vi "Autonomous Independent.vi"() -> ()   [LabVIEW 2013]
doc: "This VI is called when autonomous begins, and will automatically be terminated when autonomous ends. You can carry out timed or sensor driven robot movement independently without needing to return to the caller."
uses:
  Robot Global Data.vi
  <vilib>/Rock Robotics/WPI/RobotDrive/WPI_RobotDriveMecanumDrive_Cartesian.vi
  <vilib>/Rock Robotics/WPI/RobotDrive/WPI_RobotDriveGetSetRefNum.vi
panel:
  out "Current Movement, for debugging":T1 {"Z Joystick Value" scale=-1.0..1.0; "Y Joystick Value" scale=1.0..-1.0; "X Joystick Value" scale=-1.0..1.0}
  in  "Array of robot movements":T2(array[cluster]) {"Z Joystick Value" scale=-1.0..1.0; "Y Joystick Value" scale=1.0..-1.0; "X Joystick Value" scale=-1.0..1.0}
  # "Be sure to right-click and choose Data Operations>>Make Current Value default if you want to save the array values with the VI"
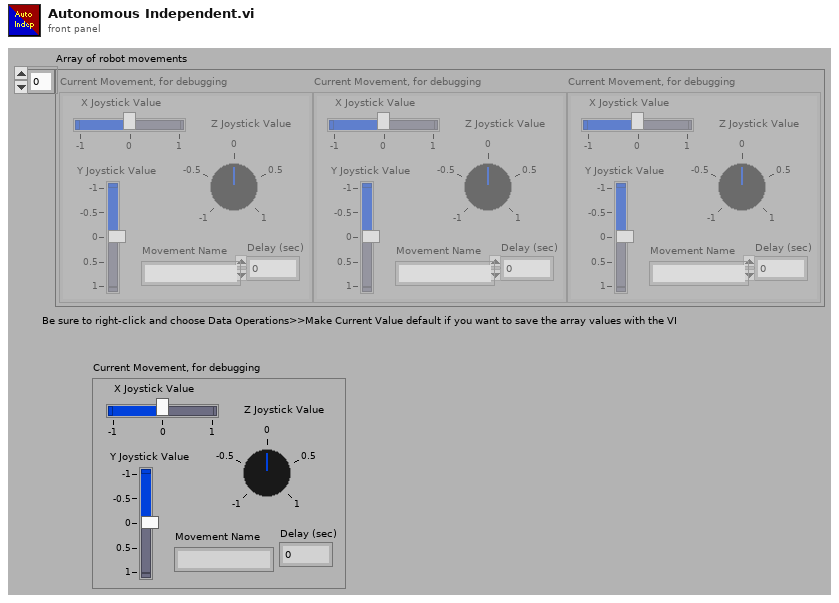
[diagram p1: front panel]
types:
  T1 = cluster{"X Joystick Value":dbl, "Y Joystick Value":dbl, "Z Joystick Value":dbl, "Delay (sec)":dbl, "Movement Name":string}
  T2 = cluster{"X Joystick Value":dbl, "Y Joystick Value":dbl, "Z Joystick Value":dbl, "Delay (sec)":dbl, "Movement Name":string}[]
  T3 = typedef "WPI_RobotDriveDevRef.ctl" = cluster{"DevStatus":errorcluster, "Motors[]":T4[], "Square Inputs":bool, "Max Output":dbl, "Isochronous":bool}
  T4 = typedef "WPI_MotorControlDeviceRef.ctl" = cluster{"DeviceStatus":errorcluster, "Type":enum16{"PWM", "CAN"}, "PWM":cluster{"Digital Module":T5, "PWM Channel":T6, "DeadBand":T7}, "CAN":cluster{"Device Number":u8, "Control Mode":T8, "Semaphore":T9, "Max Vout":dbl}, "Invert":bool, "TransformRef":T10, "InvTransformRef":T10}
  T5 = typedef "FPGA_TypedefDigitalModule.ctl" = enum16{"Digital Module 1", "Digital Module 2"}
  T6 = typedef "FPGA_DIOPWMChannel.ctl" = enum8{"PWM 1", "PWM 2", "PWM 3", "PWM 4", "PWM 5", "PWM 6", "PWM 7", "PWM 8", "PWM 9", "PWM 10", "Invalid"}
  T7 = typedef "WPI_PWMDeadband.ctl" = cluster{"Name":string, "maxPositivePwm":i32, "minPositivePwm":i32, "centerPwm":i32, "maxNegativePwm":i32, "minNegativePwm":i32, "angularRange":u16}
  T8 = typedef "WPI_CANJaguar_ControlMode.ctl" = enum8{"Percent VBus", "Current", "Speed", "Position", "Voltage"}
  T9 = typedef "Semaphore RefNum" = refnum<k1>
  T10 = typedef "WPI_PWMTransform_ConPane.ctl" = refnum<vi>
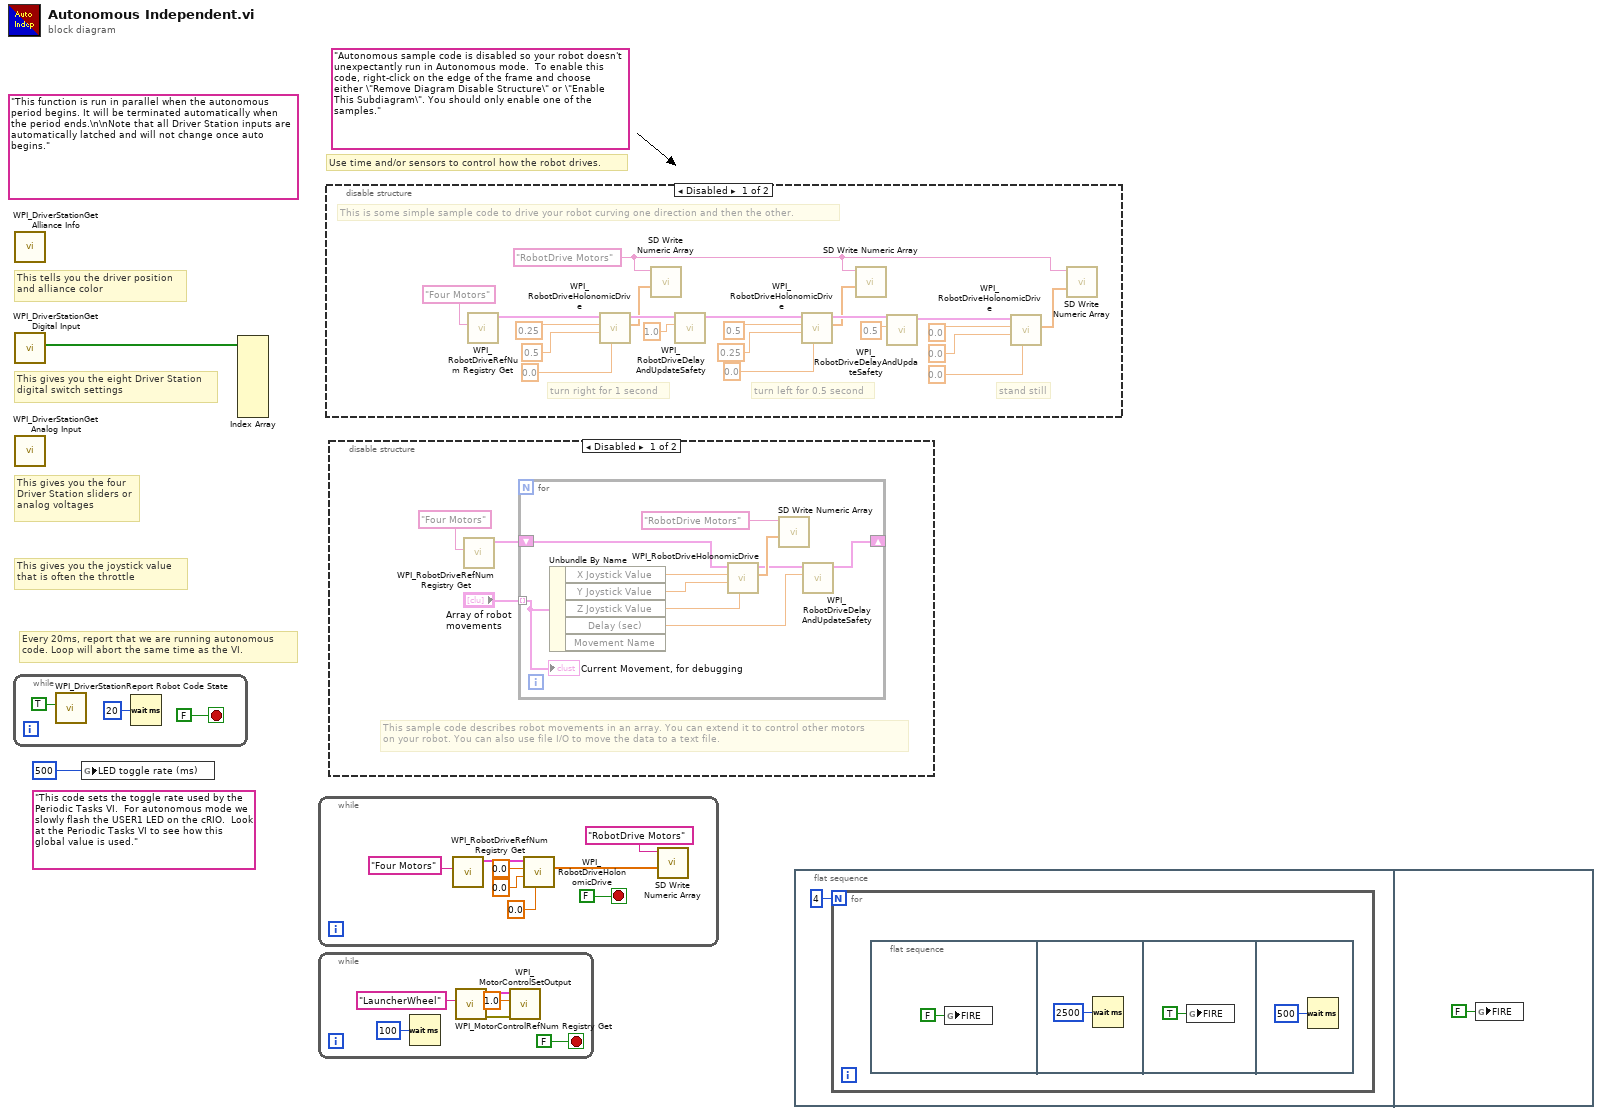
[diagram p0: block diagram]
diagram:
  (unwired) "This code sets the toggle rate used by the Periodic Tasks VI.  For autonomous mode we slowly flash the USER1 LED on the cRIO.  Look at the Periodic Tasks VI to see how this global value is used."
  (unwired) "Autonomous sample code is disabled so your robot doesn't unexpectantly run in Autonomous mode.  To enable this code, right-click on the edge of the frame and choose either \"Remove Diagram Disable Structure\" or \"Enable This Subdiagram\". You should only enable one of the samples."
  (unwired) "This function is run in parallel when the autonomous period begins. It will be terminated automatically when the period ends.\n\nNote that all Driver Station inputs are automatically latched and will not change once auto begins."
  # "Every 20ms, report that we are running autonomous\ncode. Loop will abort the same time as the VI."
  # "This gives you the joystick value\nthat is often the throttle"
  # "Use time and/or sensors to control how the robot drives."
  # "This tells you the driver position\nand alliance color"
  # "This gives you the eight Driver Station\ndigital switch settings"
  # "This gives you the four\nDriver Station sliders or\nanalog voltages"
  n1 = while {
    stop <- FALSE stop-if-true
    n2 = call <vilib>:"WPI_DriverStationReport Robot Code State.vi"("Autonomous"=TRUE) -> ()  [unwired: 10 in, 1 out]
    n3 = Wait (ms)(milliseconds to wait=u32 20) -> ()  [unwired: 1 out]
  }
  n4 = call <vilib>:"WPI_DriverStationGet Alliance Info.vi"() -> ()  [unwired: 12 out]
  n5 = call <vilib>:"WPI_DriverStationGet Digital Input.vi"() -> ("Driver Station Digital Input (1-8)"=w2:bool[])  [unwired: 11 out]
  n6 = call <vilib>:"WPI_DriverStationGet Analog Input.vi"() -> ()  [unwired: 12 out]
  n7 = global write "Robot Global Data.vi" "LED toggle rate (ms)"(u32 500 ("LED ms toggle rate")) -> ()
  n8 = Index Array(array=w2) -> ()  [unwired: 8 in, 8 out]
  n9 = while {
    stop <- FALSE stop-if-true
    n10 = call <vilib>:"WPI_RobotDriveRefNum Registry Get.vi"("refnum name"="Four Motors") -> ("RobotDriveDevRef"=w11:T3)  [unwired: 1 in, 9 out]
    n11 = call-poly <vilib>:"WPI_RobotDriveHolonomicDrive.vi"("Rotation"=0.0, "Y"=0.0, "X"=0.0, "RobotDriveDevRef"=w11) -> ("Motor Values"=w9:dbl[])  [unwired: 5 in, 2 out]
    n12 = call <vilib>:"SD Write Numeric Array.vi"("Numeric Array"=w9, "Name"="RobotDrive Motors") -> ()  [unwired: 8 in, 2 out]
  }
  n13 = while {
    stop <- FALSE stop-if-true
    n14 = Wait (ms)(milliseconds to wait=u32 100) -> ()  [unwired: 1 out]
    n15 = call <vilib>:"WPI_MotorControlRefNum Registry Get.vi"("refnum name"="LauncherWheel") -> ("error out"=w18:errorcluster, "MotorControlDevRef"=w19:T4)  [unwired: 9 in]
    n16 = call <vilib>:"WPI_MotorControlSetOutput.vi"("error in (no error)"=w18, "Output"=1.0, "MotorControlDevRef"=w19) -> ()  [unwired: 6 in, 3 out]
  }
  n17 = disable-structure shown="Disabled" {
    frame Disabled {
      w23 = "RobotDrive Motors" ("Name")
      # "This is some simple sample code to drive your robot curving one direction and then the other."
      # "stand still"
      # "turn left for 0.5 second"
      # "turn right for 1 second"
      n18 = call <vilib>:"WPI_RobotDriveRefNum Registry Get.vi"("refnum name"="Four Motors") -> ("RobotDriveDevRef"=w27:T3)  [unwired: 1 in, 9 out]
      n19 = call-poly <vilib>:"WPI_RobotDriveHolonomicDrive.vi"("Rotation"=0.0, "Y"=0.5 ("X axis value"), "X"=0.25 ("X axis value"), "RobotDriveDevRef"=w27) -> ("Motor Values"=w26:dbl[], "RobotDriveDevRef"=w34:T3)  [unwired: 5 in, 1 out]
      n20 = call <vilib>:"SD Write Numeric Array.vi"("Numeric Array"=w26, "Name"=w23) -> ()  [unwired: 8 in, 2 out]
      n21 = call <vilib>:"WPI_RobotDriveDelayAndUpdateSafety.vi"("Delay (s)"=1.0, "RobotDriveDevRef"=w34) -> ("RobotDriveDevRef 2"=w33:T3)  [unwired: 8 in, 1 out]
      n22 = call-poly <vilib>:"WPI_RobotDriveHolonomicDrive.vi"("Rotation"=0.0, "Y"=0.25 ("X axis value"), "X"=0.5 ("X axis value"), "RobotDriveDevRef"=w33) -> ("Motor Values"=w25:dbl[], "RobotDriveDevRef"=w32:T3)  [unwired: 5 in, 1 out]
      n23 = call <vilib>:"SD Write Numeric Array.vi"("Numeric Array"=w25, "Name"=w23) -> ()  [unwired: 8 in, 2 out]
      n24 = call <vilib>:"WPI_RobotDriveDelayAndUpdateSafety.vi"("Delay (s)"=0.5, "RobotDriveDevRef"=w32) -> ("RobotDriveDevRef 2"=w31:T3)  [unwired: 8 in, 1 out]
      n25 = call-poly <vilib>:"WPI_RobotDriveHolonomicDrive.vi"("Rotation"=0.0 ("X axis value"), "Y"=0.0 ("X axis value"), "X"=0.0 ("X axis value"), "RobotDriveDevRef"=w31) -> ("Motor Values"=w24:dbl[])  [unwired: 5 in, 2 out]
      n26 = call <vilib>:"SD Write Numeric Array.vi"("Numeric Array"=w24, "Name"=w23) -> ()  [unwired: 8 in, 2 out]
    }
    frame Enabled {
    }
  }
  n27 = disable-structure shown="Disabled" {
    frame Disabled {
      # "This sample code describes robot movements in an array. You can extend it to control other motors\non your robot. You can also use file I/O to move the data to a text file."
      n28 = call <vilib>:"WPI_RobotDriveRefNum Registry Get.vi"("refnum name"="Four Motors") -> ("RobotDriveDevRef"=w42:T3)  [unwired: 1 in, 9 out]
      n29 = for {
        shift-right: [w49] -> _
        shift-left: w42 -> [w50]
        tunnel: "Array of robot movements" -> [w45] mode=indexing
        n30 = Unbundle By Name(w45) -> ("X Joystick Value"=w48:dbl, "Y Joystick Value"=w47:dbl, "Z Joystick Value"=w44:dbl, "Delay (sec)"=w46:dbl)  [unwired: 1 out]
        n31 = call-poly <vilib>:"WPI_RobotDriveHolonomicDrive.vi"("Rotation"=w44, "Y"=w47, "X"=w48, "RobotDriveDevRef"=w50) -> ("Motor Values"=w52:dbl[], "RobotDriveDevRef"=w51:T3)  [unwired: 5 in, 1 out]
        n32 = call <vilib>:"SD Write Numeric Array.vi"("Numeric Array"=w52, "Name"="RobotDrive Motors") -> ()  [unwired: 8 in, 2 out]
        n33 = call <vilib>:"WPI_RobotDriveDelayAndUpdateSafety.vi"("Delay (s)"=w46, "RobotDriveDevRef"=w51) -> ("RobotDriveDevRef 2"=w49:T3)  [unwired: 8 in, 1 out]
        "Current Movement, for debugging" <- w45
      }
    }
    frame Enabled {
    }
  }
  n34 = flat-sequence {
    frame #0 {
      n35 = for {
        N: 4 -> [_]
        n36 = flat-sequence {
          frame #0 {
            n37 = global write "Robot Global Data.vi" "FIRE"(FALSE ("FIRE")) -> ()
          }
          frame #1 {
            n38 = Wait (ms)(milliseconds to wait=u32 2500) -> ()  [unwired: 1 out]
          }
          frame #2 {
            n39 = global write "Robot Global Data.vi" "FIRE"(TRUE ("FIRE")) -> ()
          }
          frame #3 {
            n40 = Wait (ms)(milliseconds to wait=u32 500) -> ()  [unwired: 1 out]
          }
        }
      }
    }
    frame #1 {
      n41 = global write "Robot Global Data.vi" "FIRE"(FALSE ("FIRE")) -> ()
    }
  }
